vi "Get Steering Type.vi"(8 "error in (no error)":errorcluster, 11 "mecanum steering frame in":refnum<class "NI_Robotics_Mecanum Steering Frame.lvclass">) -> (0 "error out":errorcluster, 2 "steering type":string, 3 "mecanum steering frame out":refnum<class "NI_Robotics_Mecanum Steering Frame.lvclass">)   [LabVIEW 2017, in "NI_Robotics_Mecanum Steering Frame.lvclass"]
uses:
  <vilib>/robotics/Steering/Mecanum Steering Frame/NI_Robotics_Mecanum Steering Frame.lvclass
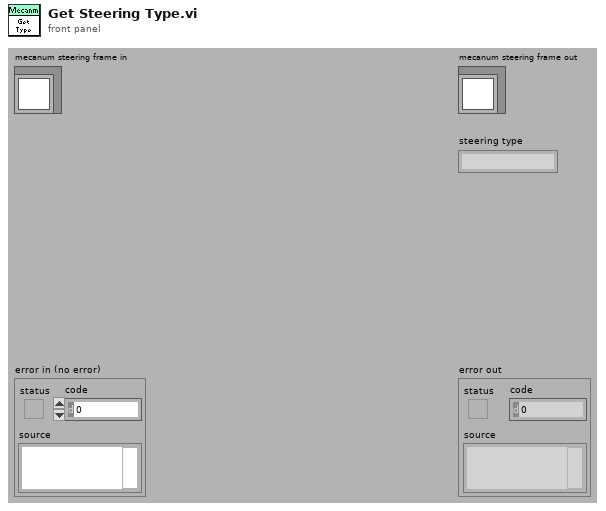
[diagram p1: front panel]
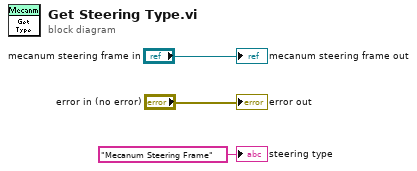
[diagram p0: block diagram]
diagram:
  "error out" <- "error in (no error)"
  "mecanum steering frame out" <- "mecanum steering frame in"
  "steering type" <- "Mecanum Steering Frame" ("Steering Type")
